vi "GroundStation final.vi"() -> ()   [LabVIEW 2022 SP3]
uses:
  <vilib>/Instr/_visa.llb/VISA Configure Serial Port (Instr).vi
  <vilib>/Utility/file.llb/Write Delimited Spreadsheet (string).vi
  <vilib>/picture/3D Picture Control/Object/Create Object (name).vi
  <vilib>/picture/3D Picture Control/Object/Add Object (no reference).vi
  <vilib>/picture/3D Picture Control/NI_3D Picture Control.lvlib
  <vilib>/httpClient/LabVIEWHTTPClient.lvlib
panel:
  out "Gas 3":string="Kg/M^3"
  out "Gas 2":dbl caption="Gas"
  out "X_axis 2":string
  out "Z_axis 2":string
  out "LiDAR_Read":string
  out "Angle":string
  out "Y_axis":string
  out "MPU 2":string
  out "GPS 3":string
  out "ANGLE Z":dbl
  out "ANGLE Y":dbl
  out "ANGLE X":dbl
  out "BMP 2":string
  out "MQ 2":string
  out "LIDAR":string
  out "Space":string
  out "DHT":string
  out "SPACE":string
  out "TEMP":string
  out "RH":string
  out "ALTITUDE":string
  out "PRESSURE":string
  out "GAS":string
  in  "Tab Control 2":enum32{"DASHBOARD", "SENSORS", "ABOUT"}(tab)
  out "Low Power":bool
  out "DHT":bool
  out "BMP":bool
  out "MQ":bool
  out "LIDAR":bool
  out "MPU":bool
  out "Pressure  2":dbl caption="Pressure"
  out "Pressure":string="Pascal"
  out "Altitude":string="Km/S^2"
  out "Altitude 2":dbl caption="Gas"
  out "Humidity":string="Km/S^2"
  out "rh":dbl caption="Humidity"
  out "Temp.":string="Celsius"
  out "Temperture 2":dbl caption="Temp"
  out "GPS":bool
  in  "Save Button":bool
  in  "Media Stop Button":bool
  in  "Play Button":bool
  out "System Status":string
  out "Battery Precentage":dbl format="%%%#_g"
  in  "Set Mode Button":bool
  in  "System Mode":T1(ring)
  in  "Save File Path":path
  in  "VISA resource name":refnum<visa-resource-name>
  in  "Save Button 2":bool
  out "Massage":string
  in  "Tab Control 4":T2(tab) caption="Tab Control 3"
  out "YAW":string
  out "PITCH":string
  out "ROLL":string
  out "Z MPU":string
  out "Y MPU":string
  out "X MPU":string
  in  "File Path":path
  in  "Apply Filter":bool
  out "Waveform Chart":dynamicdata(graph)
  out "3D Picture 2":refnum<vi>(3d-picture)
  out "z_axis":dbl
  out "Y_axis":dbl
  out "X_axis":dbl
  out "LIDAR_Read":dbl
  out "ANGLE":dbl
  out "XY Graph":cluster{"Y":dbl[], "Y":dbl[]}[](graph)
  out "Camera View":T3(plugin-control)
  in  "Stop Camera":bool
  in  "Start Camera":bool
  in  "Size Y":dbl
  in  "Size X":dbl
  in  "Zoom":dbl
  in  "Map Format":string(combo)
  in  "Character":string
  in  "Color":string
  in  "WebBrowser":refnum<k7>(container)
  out "LATITUDE":string
  out "LONGTUDE":string
  # "EARTH OBSERVATION SATELITE 2025"
  # "Power Management"
  # "Warnings"
  # "Live Sensors"
  # "Quick Actions"
  # "IMU & Orientation"
  # "This interface is part of a student project to develop a Ground Station for monitoring a CubeSat. It displays real-time sensor data, manages power modes, and streams live video from the satellite."
  # "Developed by:\n\n  Nevin Essam Helmy Gaber\n Youssif Ashraf \n\nAlong With the Team Members: \n\n Maged Micheal Seha     \n Abd-Elrahman Ramadan   \n Rawan Wael Elsayed   \n Bassam Khaled Eldawy  \n Marwa Gamal Hendawy    \n Yomna Saad Abd-Elazeem  \n Bavly Emil Tamer   \n Mostafa Mohamed Tawfik   \n Mariam Emadeldin Abdelrazik  \n Maryam Reda Elsayed   \n\nContact US:\n +201204037805"
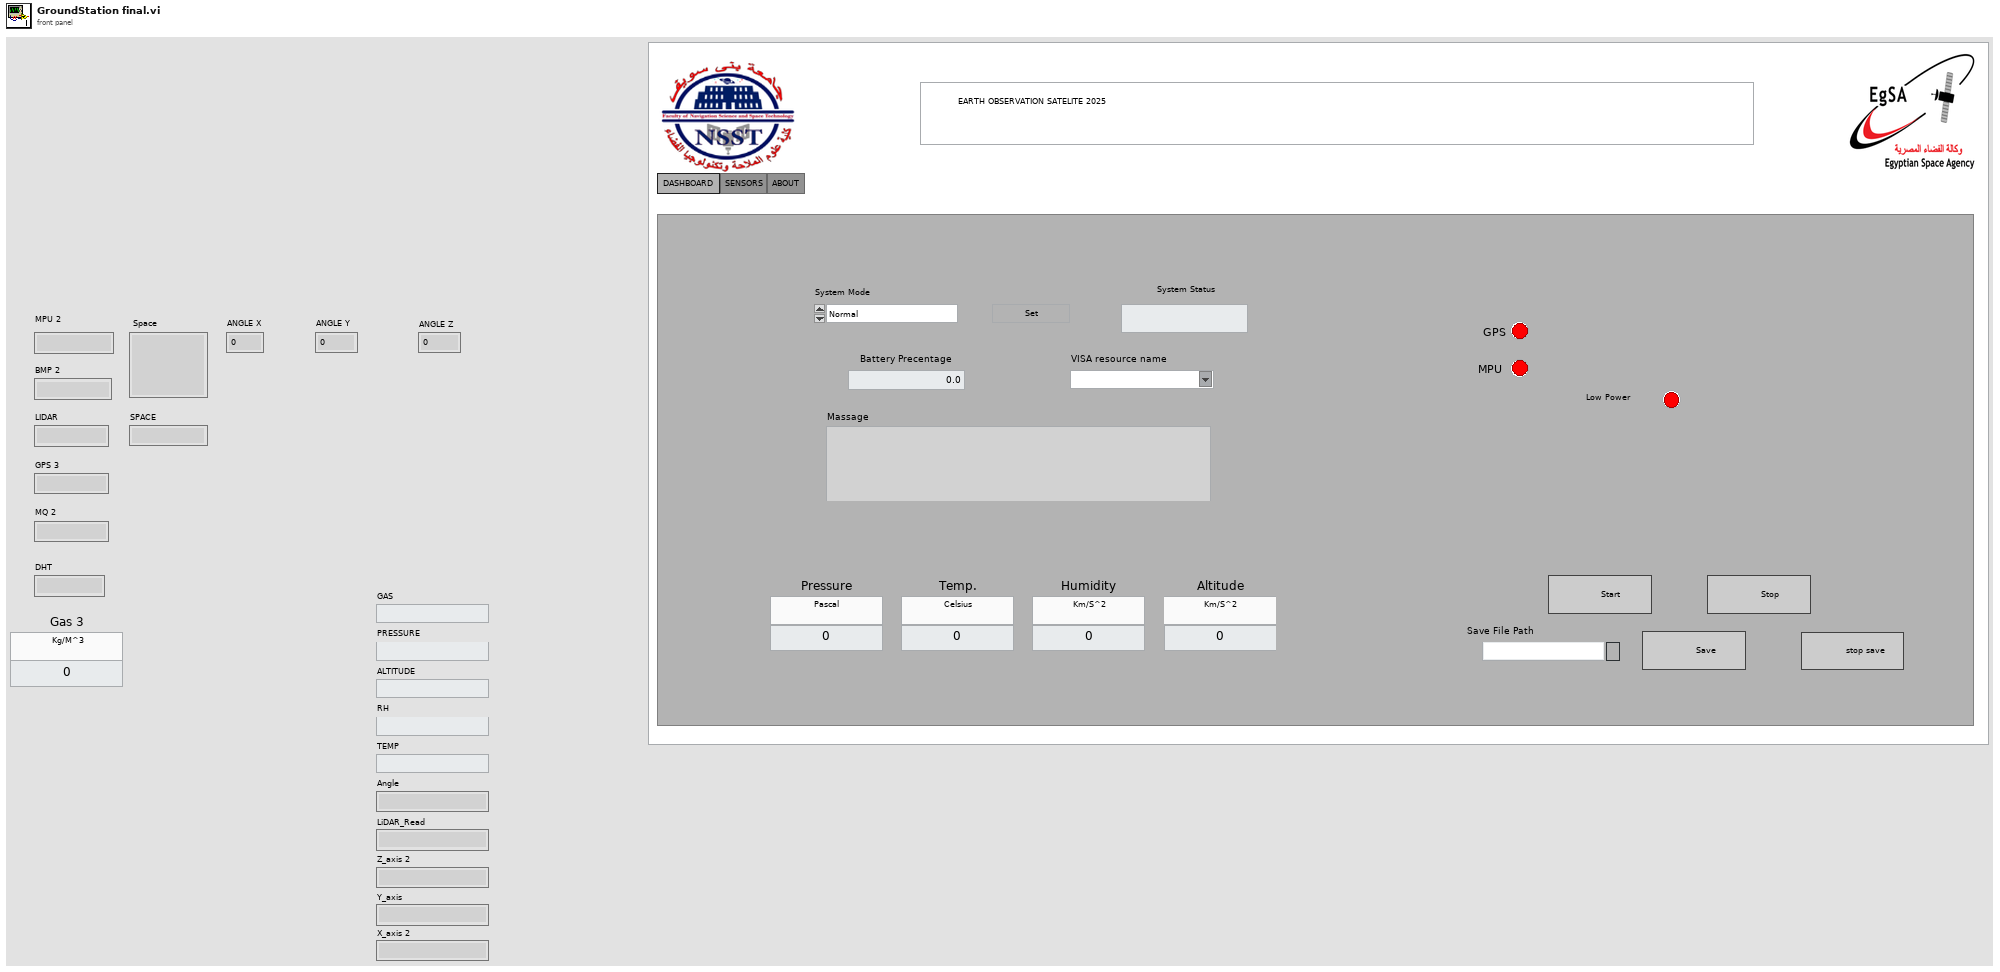
[diagram p1: front panel]
types:
  T1 = enum16{"Normal", "Power Saving", "Emergency", "Sleep"}
  T2 = enum32{"Sensors", "Sensors 2", "Ranging & Nav", "Vision & AI"}
  T3 = typedef "IMAQ Image.ctl" = refnum<image>
  T4 = typedef "Image Type" = u32
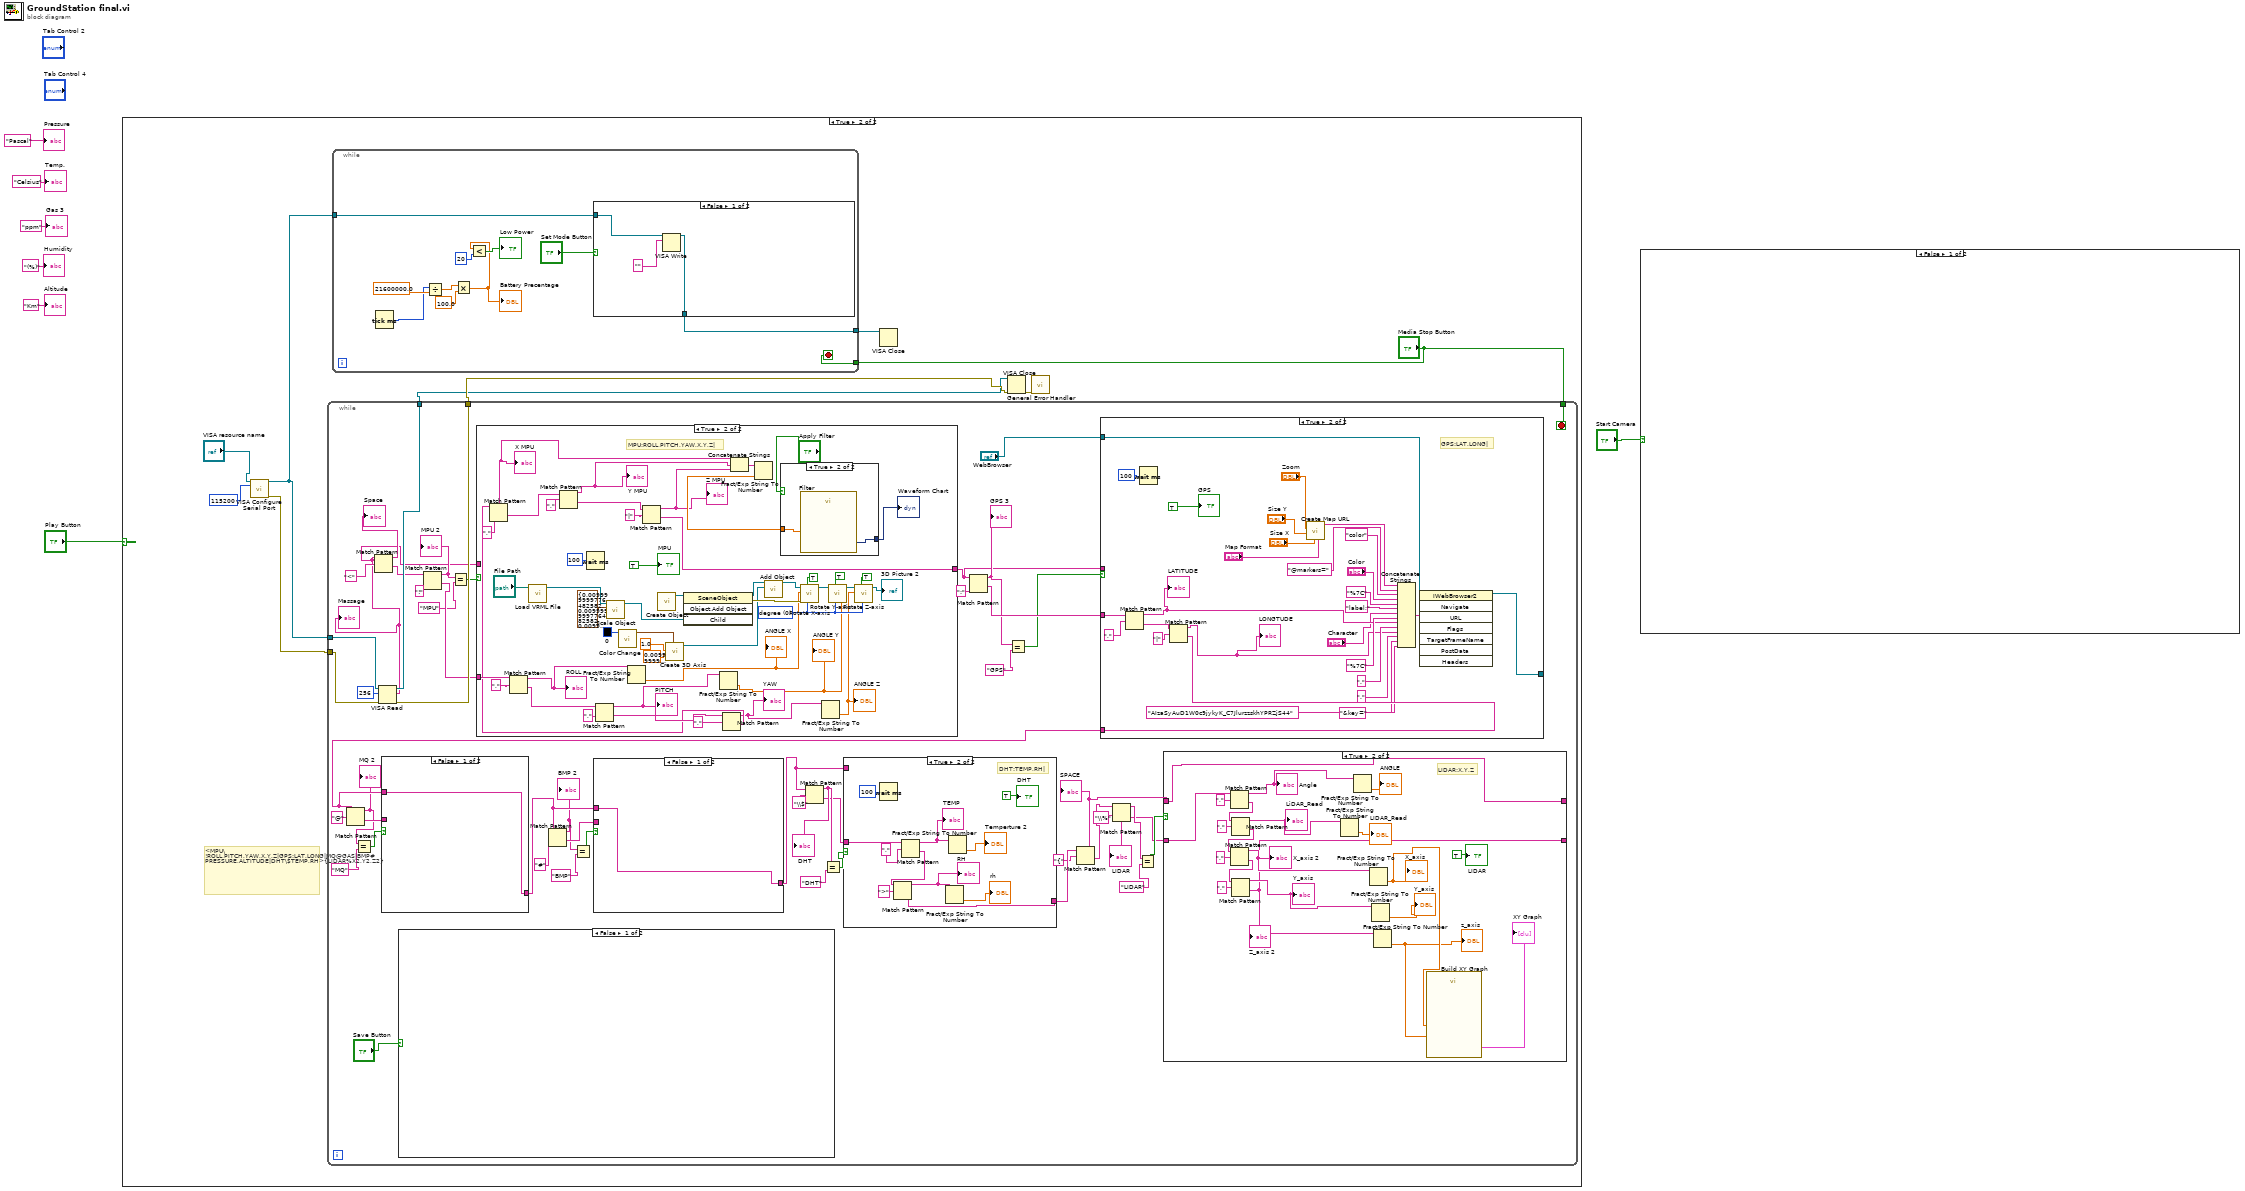
[diagram p0: block diagram]
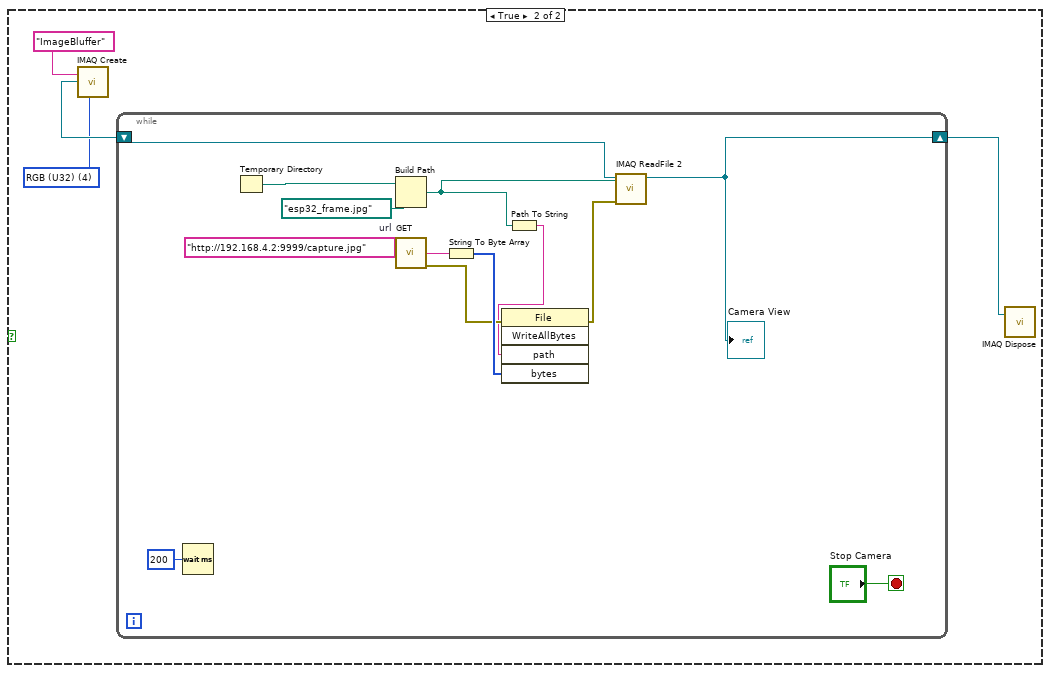
[diagram p2: hidden frame]
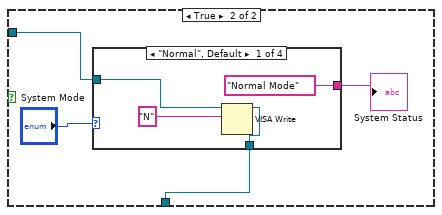
[diagram p4: hidden frame]
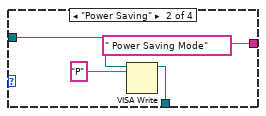
[diagram p5: hidden frame]
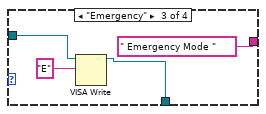
[diagram p6: hidden frame]
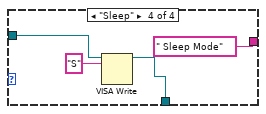
[diagram p7: hidden frame]
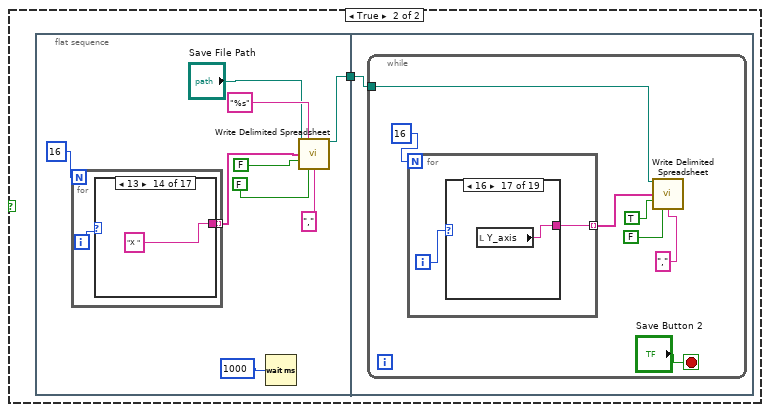
[diagram p8: hidden frame]
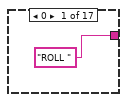
[diagram p9: hidden frame]
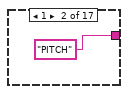
[diagram p10: hidden frame]
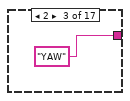
[diagram p11: hidden frame]
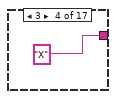
[diagram p12: hidden frame]
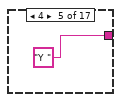
[diagram p13: hidden frame]
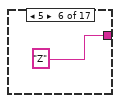
[diagram p14: hidden frame]
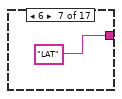
[diagram p15: hidden frame]
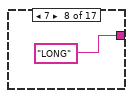
[diagram p16: hidden frame]
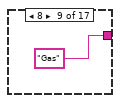
[diagram p17: hidden frame]
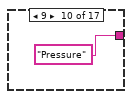
[diagram p18: hidden frame]
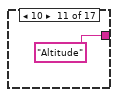
[diagram p19: hidden frame]
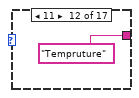
[diagram p20: hidden frame]
diagram:
  n1 = case shown="True" "Play Button" {
    frame False {
    }
    frame True {
      # "<MPU\\!ROLL,PITCH,YAW,X,Y,Z|GPS:LAT,LONG|MQ@GAS|BMP#PRESSURE,ALTITUDE|DHT\\$TEMP,RH>{LIDAR%X2,Y2,Z2}"
      n2 = call-poly "VISA Configure Serial Port"("VISA resource name"="VISA resource name", "baud rate (9600)"=u32 115200) -> ("VISA resource name out"=w9:refnum<visa-resource-name>, "error out"=w13:errorcluster)  [unwired: 12 in]
      n3 = while {
        tunnel: w9 -> [w100]
        tunnel: [w99] -> w15
        tunnel: w13 -> [w90]
        tunnel: [w91] -> w16
        tunnel: "Media Stop Button" -> [w59]
        stop <- w59 stop-if-true
        n4 = VISA Read(VISA resource name=w100, byte count=u32 256, error in (no error)=w90) -> (VISA resource name out=w99:refnum<visa-resource-name>, read buffer=w52:string, error out=w91:errorcluster)  [unwired: 1 out]
        "Massage" <- w52
        n5 = Match Pattern(string=w52, regular expression="<") -> (before substring=→"Space":string, after substring=w62:string)  [unwired: 1 in, 2 out]
        n6 = case shown="False" "Save Button" {
          frame False {
          }
          frame True {
            n7 = flat-sequence {
              tunnel: [w106] -> w101
              tunnel: w101 -> [w129]
              frame #0 {
                n8 = for {
                  N: 16 -> [_]
                  tunnel: [w111] -> w103 mode=indexing
                  i -> [w112]
                  n9 = case shown="13" w112 {
                    tunnel: ["ROLL " "PITCH" "YAW" "X" "Y " "Z" "LAT" "LONG" "Gas" "Pressure" "Altitude" "Tempruture" "RH " "X " "Y " "Z " _] -> w111
                    frame 0 {
                    }
                    frame 1 {
                    }
                    frame 2 {
                    }
                    frame 3 {
                    }
                    frame 4 {
                    }
                    frame 5 {
                    }
                    frame 6 {
                    }
                    frame 7 {
                    }
                    frame 8 {
                    }
                    frame 9 {
                    }
                    frame 10 {
                    }
                    frame 11 {
                    }
                    frame 12 {
                    }
                    frame 13 {
                    }
                    frame 14 {
                    }
                    frame 15 {
                    }
                    frame Default {
                    }
                  }
                }
                n10 = Wait (ms)(milliseconds to wait=u32 1000) -> ()  [unwired: 1 out]
                n11 = call-poly <vilib>:"Write Delimited Spreadsheet.vi"("file path (dialog if empty)"="Save File Path", "format (%s)"="%s" ("format (%.3f)"), "1D data"=w103, "append to file? (new file:F)"=FALSE, "transpose? (no:F)"=FALSE, "delimiter (\\t)"="," ("delimiter (\\t)")) -> ("new file path (Not A Path if cancelled)"=w106:path)  [unwired: 8 in, 1 out]
              }
              frame #1 {
                n12 = while {
                  tunnel: w129 -> [w132]
                  stop <- "Save Button 2" stop-if-true
                  n13 = for {
                    N: 16 -> [_]
                    tunnel: [w138] -> w131 mode=indexing
                    i -> [w137]
                    n14 = case shown="16" w137 {
                      tunnel: [w139 w140 w141 w142 w143 w144 w145 w146 w147 w148 w149 w150 w151 w152 w153 w154 w155 w156 _] -> w138
                      frame 0 {
                        n15 = local read "ROLL"() -> (w139:string)
                      }
                      frame 1 {
                        n16 = local read "PITCH"() -> (w140:string)
                      }
                      frame 2 {
                        n17 = local read "YAW"() -> (w141:string)
                      }
                      frame 3 {
                        n18 = local read "X MPU"() -> (w142:string)
                      }
                      frame 4 {
                        n19 = local read "Y MPU"() -> (w143:string)
                      }
                      frame 5 {
                        n20 = local read "Z MPU"() -> (w144:string)
                      }
                      frame 6 {
                        n21 = local read "LATITUDE"() -> (w145:string)
                      }
                      frame 7 {
                        n22 = local read "LONGTUDE"() -> (w146:string)
                      }
                      frame 8 {
                        n23 = local read "GAS"() -> (w147:string)
                      }
                      frame 9 {
                        n24 = local read "PRESSURE"() -> (w148:string)
                      }
                      frame 10 {
                        n25 = local read "ALTITUDE"() -> (w149:string)
                      }
                      frame 11 {
                        n26 = local read "TEMP"() -> (w150:string)
                      }
                      frame 12 {
                        n27 = local read "RH"() -> (w151:string)
                      }
                      frame 13 {
                        n28 = local read "Angle"() -> (w152:string)
                      }
                      frame 14 {
                        n29 = local read "LiDAR_Read"() -> (w153:string)
                      }
                      frame 15 {
                        n30 = local read "X_axis 2"() -> (w154:string)
                      }
                      frame 16 {
                        n31 = local read "Y_axis"() -> (w155:string)
                      }
                      frame 17 {
                        n32 = local read "Z_axis 2"() -> (w156:string)
                      }
                      frame 18, Default {
                      }
                    }
                  }
                  n33 = call-poly <vilib>:"Write Delimited Spreadsheet.vi"("file path (dialog if empty)"=w132, "1D data"=w131, "append to file? (new file:F)"=TRUE, "transpose? (no:F)"=FALSE, "delimiter (\\t)"="," ("delimiter (\\t)")) -> ()  [unwired: 9 in, 2 out]
                }
              }
            }
          }
        }
        n34 = Match Pattern(string=w62, regular expression="!") -> (before substring=w81:string, after substring=w89:string)  [unwired: 1 in, 2 out]
        "MPU 2" <- w81
        n35 = Equal?(x=w81, y="MPU") -> (x = y?=w83:bool)
        n36 = case shown="True" w83 {
          tunnel: w89 -> [_ w290]
          tunnel: [w242 w243] -> w51
          tunnel: w52 -> [w242 _]
          frame False {
          }
          frame True {
            w279 = u16 0 items=["degree", "radians"] ("angle unit")
            # "MPU:ROLL,PITCH,YAW,X,Y,Z|"
            n37 = Match Pattern(string=w290, regular expression=",") -> (before substring=w248:string, after substring=w261:string)  [unwired: 1 in, 2 out]
            "ROLL" <- w248
            n38 = call <vilib>:"Load VRML File.vi"("Path"="File Path") -> ("Scene:Read Scene File"=w265:refnum<vi>)  [unwired: 9 in, 1 out]
            n39 = Wait (ms)(milliseconds to wait=u32 100 ("millisecond timer value")) -> ()  [unwired: 1 out]
            n40 = Match Pattern(string=w261, regular expression=",") -> (before substring=w245:string, after substring=w260:string)  [unwired: 1 in, 2 out]
            "PITCH" <- w245
            n41 = call <vilib>:"Scale Object.vi"("Scale"=cluster{"X":sgl, "Y":sgl, "Z":sgl} {"X"=0.01, "Y"=0.01, "Z"=0.01}, "Scene.Object In"=w265) -> ("Scene.Object Out"=w264:refnum<vi>)  [unwired: 8 in, 1 out]
            n42 = call <vilib>:"Color Change.vi"("Color"=u32 0 ("Color Box")) -> ("RGBA"=w268:cluster{"R":sgl, "G":sgl, "B":sgl, "A":sgl})  [unwired: 10 in]
            n43 = Fract/Exp String To Number(string=w248) -> (number=w255:dbl)  [unwired: 3 in, 1 out]
            "ANGLE X" <- w255
            n44 = call-poly <vilib>:"Create Object.vi"() -> ("Scene:New Object"=w267:refnum<vi>)  [unwired: 10 in, 1 out]
            n45 = call <vilib>:"Create 3D Axis.vi"("Color"=w268, "Radius"=sgl 0.01, "Length"=sgl 1.0) -> ("New Object Refnum"=w283:refnum<vi>)  [unwired: 7 in, 1 out]
            n46 = invoke class="SceneObject" method="Object.Add Object"(reference=w267, "Child"=w264) -> (reference out=w284:refnum<vi>, error out=w288:errorcluster)  [unwired: 2 in, 2 out]
            n47 = Fract/Exp String To Number(string=w245) -> (number=w256:dbl)  [unwired: 3 in, 1 out]
            "ANGLE Y" <- w256
            n48 = Match Pattern(string=w260, regular expression=",") -> (before substring=w247:string, after substring=w259:string)  [unwired: 1 in, 2 out]
            "YAW" <- w247
            n49 = Match Pattern(string=w259, regular expression=",") -> (before substring=w254:string, after substring=w270:string)  [unwired: 1 in, 2 out]
            "X MPU" <- w254
            n50 = Match Pattern(string=w270, regular expression=",") -> (before substring=w244:string, after substring=w269:string)  [unwired: 1 in, 2 out]
            "Y MPU" <- w244
            n51 = Match Pattern(string=w269, regular expression="|") -> (before substring=w253:string, after substring=w243:string)  [unwired: 1 in, 2 out]
            "Z MPU" <- w253
            n52 = Concatenate Strings(w254, w244, w253) -> (w263:string)
            n53 = Fract/Exp String To Number(string=w263) -> (number=w289:dbl)  [unwired: 3 in, 1 out]
            n54 = call-poly <vilib>:"Add Object.vi"("New Object In"=w283, "Scene Object In"=w284) -> ("Scene Object Out"=w282:refnum<vi>)  [unwired: 8 in, 1 out]
            n55 = case shown="True" "Apply Filter" {
              tunnel: w289 -> [_ w292]
              tunnel: [w291 w293] -> w252
              frame False {
                n56 = call "Convert to Dynamic Data"() -> ("Dynamic Data Type"=w291:dynamicdata)  [unwired: 4 in]
              }
              frame True {
                n57 = call "Filter"("Signal"=w292) -> ("Filtered Signal"=w293:dynamicdata)  [unwired: 9 in, 1 out]
              }
            }
            "Waveform Chart" <- w252
            n58 = call <vilib>:"Rotate X-axis.vi"("angle unit"=w279, "Relative?"=TRUE, "error in (no error)"=w288, "angle"=w255, "Scene Object In"=w282) -> ("Scene Object Out"=w281:refnum<vi>)  [unwired: 5 in, 1 out]
            n59 = Fract/Exp String To Number(string=w247) -> (number=w257:dbl)  [unwired: 3 in, 1 out]
            "ANGLE Z" <- w257
            n60 = call <vilib>:"Rotate Y-axis.vi"("angle unit"=w279, "Relative?"=TRUE, "angle"=w256, "Scene Object In"=w281) -> ("Scene Object Out"=w280:refnum<vi>)  [unwired: 6 in, 1 out]
            n61 = call <vilib>:"Rotate Z-axis.vi"("angle unit"=w279, "Relative?"=TRUE, "angle"=w257, "Scene Object In"=w280) -> ("Scene Object Out"=→"3D Picture 2":refnum<vi>)  [unwired: 6 in, 1 out]
            "MPU" <- TRUE
          }
        }
        n62 = Match Pattern(string=w51, regular expression=":") -> (before substring=w79:string, after substring=w88:string)  [unwired: 1 in, 2 out]
        "GPS 3" <- w79
        n63 = Equal?(x=w79, y="GPS") -> (x = y?=w78:bool)
        n64 = case shown="True" w78 {
          tunnel: "WebBrowser" -> [w213 w241]
          tunnel: [w212 w240] -> w84
          tunnel: w88 -> [_ w239]
          tunnel: [w213 w223] -> _
          tunnel: w51 -> [w212 _]
          frame False {
          }
          frame True {
            # "GPS:LAT,LONG|"
            n65 = Match Pattern(string=w239, regular expression=",") -> (before substring=w221:string, after substring=w225:string)  [unwired: 1 in, 2 out]
            "LATITUDE" <- w221
            n66 = Wait (ms)(milliseconds to wait=u32 100) -> ()  [unwired: 1 out]
            n67 = Match Pattern(string=w225, regular expression="|") -> (before substring=w220:string, after substring=w240:string)  [unwired: 1 in, 2 out]
            "LONGTUDE" <- w220
            n68 = call "Create Map URL.vi"("Map Format"="Map Format", "X"="Size X", "Y"="Size Y", "Zoom"="Zoom") -> ("String"=w238:string)  [unwired: 7 in]
            n69 = Concatenate Strings(w238, "@markers=" ("string"), "color" ("string"), "Color", "%7C" ("string"), "label;" ("string"), "Character", "%7C" ("string"), w221, "." ("string"), w220, "." ("string"), "&key=" ("string"), "AIzaSyAuD1W0c9jykyK_C7JlurzzskhYPRZjS44" ("string")) -> (w232:string)
            n70 = invoke class="IWebBrowser2" method="Navigate"(reference=w241, "URL"=w232) -> (reference out=w223:refnum<k7>)  [unwired: 6 in, 7 out]
            "GPS" <- TRUE
          }
        }
        n71 = Match Pattern(string=w84, regular expression="@") -> (before substring=w76:string, after substring=w87:string)  [unwired: 1 in, 2 out]
        "MQ 2" <- w76
        n72 = Equal?(x=w76, y="MQ") -> (x = y?=w75:bool)
        n73 = case shown="False" w75 {
          tunnel: w87 -> [_ w211]
          tunnel: [w204 w210] -> w85
          tunnel: w84 -> [w204 _]
          frame False {
          }
          frame True {
            # "MQ:GAS|"
            n74 = Match Pattern(string=w211, regular expression="|") -> (before substring=w205:string, after substring=w210:string)  [unwired: 1 in, 2 out]
            "GAS" <- w205
            n75 = Wait (ms)(milliseconds to wait=u32 100) -> ()  [unwired: 1 out]
            n76 = Fract/Exp String To Number(string=w205) -> (number=→"Gas 2":dbl)  [unwired: 3 in, 1 out]
            "MQ" <- TRUE
          }
        }
        n77 = Match Pattern(string=w85, regular expression="#") -> (before substring=w73:string, after substring=w86:string)  [unwired: 1 in, 2 out]
        "BMP 2" <- w73
        n78 = Equal?(x=w73, y="BMP") -> (x = y?=w72:bool)
        n79 = case shown="False" w72 {
          tunnel: [w192 w203] -> w64
          tunnel: w86 -> [_ w202]
          tunnel: w85 -> [w192 _]
          frame False {
          }
          frame True {
            # "BMP:PRESSURE,ALTITUDE|"
            n80 = Wait (ms)(milliseconds to wait=u32 100) -> ()  [unwired: 1 out]
            n81 = Match Pattern(string=w202, regular expression=",") -> (before substring=w196:string, after substring=w198:string)  [unwired: 1 in, 2 out]
            "PRESSURE" <- w196
            n82 = Match Pattern(string=w198, regular expression="|") -> (before substring=w194:string, after substring=w203:string)  [unwired: 1 in, 2 out]
            "ALTITUDE" <- w194
            n83 = Fract/Exp String To Number(string=w196) -> (number=→"Pressure  2":dbl)  [unwired: 3 in, 1 out]
            n84 = Fract/Exp String To Number(string=w194) -> (number=→"Altitude 2":dbl)  [unwired: 3 in, 1 out]
            "BMP" <- TRUE
          }
        }
        n85 = Match Pattern(string=w64, regular expression="\\$") -> (before substring=w66:string, after substring=w65:string)  [unwired: 1 in, 2 out]
        "DHT" <- w66
        n86 = Equal?(x=w66, y="DHT") -> (x = y?=w70:bool)
        n87 = case shown="True" w70 {
          tunnel: w65 -> [_ w191]
          tunnel: [w180 w190] -> w61
          tunnel: w64 -> [w180 _]
          frame False {
          }
          frame True {
            # "DHT:TEMP,RH|"
            n88 = Wait (ms)(milliseconds to wait=u32 100) -> ()  [unwired: 1 out]
            n89 = Match Pattern(string=w191, regular expression=",") -> (before substring=w183:string, after substring=w186:string)  [unwired: 1 in, 2 out]
            "TEMP" <- w183
            n90 = Match Pattern(string=w186, regular expression=">") -> (before substring=w181:string, after substring=w190:string)  [unwired: 1 in, 2 out]
            "RH" <- w181
            n91 = Fract/Exp String To Number(string=w181) -> (number=→"rh":dbl)  [unwired: 3 in, 1 out]
            n92 = Fract/Exp String To Number(string=w183) -> (number=→"Temperture 2":dbl)  [unwired: 3 in, 1 out]
            "DHT" <- TRUE
          }
        }
        n93 = Match Pattern(string=w61, regular expression="{") -> (before substring=w54:string, after substring=w55:string)  [unwired: 1 in, 2 out]
        "SPACE" <- w54
        n94 = Match Pattern(string=w55, regular expression="\\%") -> (before substring=w68:string, after substring=w56:string)  [unwired: 1 in, 2 out]
        "LIDAR" <- w68
        n95 = Equal?(x=w68, y="LIDAR") -> (x = y?=w67:bool)
        n96 = case shown="True" w67 {
          tunnel: w56 -> [w157 w171]
          tunnel: [w158 w163] -> _
          tunnel: w54 -> [w158 w163]
          tunnel: [w157 w164] -> _
          frame False {
          }
          frame True {
            # "LIDAR:X,Y,Z"
            n97 = Match Pattern(string=w171, regular expression=",") -> (before substring=w170:string, after substring=w174:string)  [unwired: 1 in, 2 out]
            "Angle" <- w170
            n98 = Match Pattern(string=w174, regular expression=",") -> (before substring=w168:string, after substring=w172:string)  [unwired: 1 in, 2 out]
            "LiDAR_Read" <- w168
            n99 = Match Pattern(string=w172, regular expression=",") -> (before substring=w167:string, after substring=w173:string)  [unwired: 1 in, 2 out]
            "X_axis 2" <- w167
            n100 = Match Pattern(string=w173, regular expression=",") -> (before substring=w165:string, after substring=w164:string)  [unwired: 1 in, 2 out]
            "Y_axis" <- w165
            "Z_axis 2" <- w164
            n101 = Fract/Exp String To Number(string=w168) -> (number=→"LIDAR_Read":dbl)  [unwired: 3 in, 1 out]
            n102 = Fract/Exp String To Number(string=w170) -> (number=→"ANGLE":dbl)  [unwired: 3 in, 1 out]
            n103 = Fract/Exp String To Number(string=w167) -> (number=w160:dbl)  [unwired: 3 in, 1 out]
            "X_axis" <- w160
            n104 = Fract/Exp String To Number(string=w165) -> (number=→"Y_axis":dbl)  [unwired: 3 in, 1 out]
            n105 = Fract/Exp String To Number(string=w164) -> (number=w159:dbl)  [unwired: 3 in, 1 out]
            "z_axis" <- w159
            n106 = call "Build XY Graph"("Y Input"=w159, "X Input"=w160) -> ("XY Graph"=→"XY Graph":cluster{"X":dbl[], "Y":dbl[]}[])  [unwired: 8 in, 1 out]
            "LIDAR" <- TRUE
          }
        }
      }
      n107 = while {
        tunnel: "Media Stop Button" -> [w24]
        tunnel: w9 -> [w23]
        tunnel: [w18] -> w8
        stop <- w24 stop-if-true
        n108 = Tick Count (ms)() -> (millisecond timer value=w17:u32)
        n109 = Divide(x=w17, y=21600000.0) -> (x/y=w21:dbl)
        n110 = Multiply(x=w21, y=100.0) -> (x*y=w19:dbl)
        "Battery Precentage" <- w19
        n111 = Less?(x=w19, y=20) -> (x < y?=→"Low Power":bool)
        n112 = case shown="False" "Set Mode Button" {
          tunnel: w23 -> [w29 w32]
          tunnel: [w28 w31] -> w18
          frame False {
            n113 = VISA Write(VISA resource name=w29, write buffer="") -> (VISA resource name out=w28:refnum<visa-resource-name>)  [unwired: 1 in, 2 out]
          }
          frame True {
            n114 = case shown="\"Normal\", Default" "System Mode" {
              tunnel: ["Normal Mode" " Power Saving Mode" " Emergency Mode " " Sleep Mode"] -> w33
              tunnel: w32 -> [w36 w40 w44 w48]
              tunnel: [w35 w39 w43 w47] -> w31
              frame "Normal", Default {
                n115 = VISA Write(VISA resource name=w36, write buffer="N") -> (VISA resource name out=w35:refnum<visa-resource-name>)  [unwired: 1 in, 2 out]
              }
              frame "Power Saving" {
                n116 = VISA Write(VISA resource name=w40, write buffer="P") -> (VISA resource name out=w39:refnum<visa-resource-name>)  [unwired: 1 in, 2 out]
              }
              frame "Emergency" {
                n117 = VISA Write(VISA resource name=w44, write buffer="E") -> (VISA resource name out=w43:refnum<visa-resource-name>)  [unwired: 1 in, 2 out]
              }
              frame "Sleep" {
                n118 = VISA Write(VISA resource name=w48, write buffer="S") -> (VISA resource name out=w47:refnum<visa-resource-name>)  [unwired: 1 in, 2 out]
              }
            }
            "System Status" <- w33
          }
        }
      }
      n119 = VISA Close(VISA resource name=w8) -> ()  [unwired: 1 in, 1 out]
      n120 = VISA Close(VISA resource name=w15, error in (no error)=w16) -> (error out=w14:errorcluster)
      n121 = call <vilib>:"General Error Handler.vi"("error in (no error)"=w14) -> ()  [unwired: 10 in, 5 out]
    }
  }
  n122 = case shown="False" "Start Camera" {
    frame False {
    }
    frame True {
      w295 = T4 4 items=["Grayscale (U8)", "Grayscale (I16)", "Grayscale (SGL)", "Complex (CSG)", "RGB (U32)", "HSL (U32)", "RGB (U64)", "Grayscale (U16)"] ("Image Type")
      n123 = call "IMAQ Create"("Image Name"="ImageBluffer", "Image Type"=w295) -> ("New Image"=w296:T3)  [unwired: 3 in, 1 out]
      n124 = while {
        shift-right: [w299] -> w294
        shift-left: w296 -> [w309]
        stop <- "Stop Camera" stop-if-true
        w310 = "http://192.168.4.2:9999/capture.jpg"  # url
        n125 = Wait (ms)(milliseconds to wait=u32 200) -> ()  [unwired: 1 out]
        n126 = Temporary Directory() -> (w308:path)
        n127 = Build Path(base path=w308, name or relative path=path "esp32_frame.jpg") -> (appended path=w301:path)
        n128 = call <vilib>:"GET.vi"("url"=w310) -> ("body"=w305:string, "error out"=w303:errorcluster)  [unwired: 11 in, 2 out]
        n129 = String To Byte Array(string=w305) -> (unsigned byte array=w304:u8[])
        n130 = Path To String(path=w301) -> (string=w300:string)
        n131 = invoke class="File" method="WriteAllBytes"(error in=w303, "path"=w300, "bytes"=w304) -> (error out=w302:errorcluster)  [unwired: 2 in, 4 out]
        n132 = call "IMAQ ReadFile 2"("File Path"=w301, "error in (no error)"=w302, "Image"=w309) -> ("Image Out"=w299:T3)  [unwired: 4 in, 4 out]
        "Camera View" <- w299
      }
      n133 = call "IMAQ Dispose"("Image"=w294) -> ()  [unwired: 5 in, 1 out]
    }
  }
  "Pressure" <- "Pascal" ("Pressure")
  "Temp." <- "Celsius" ("Temp.")
  "Gas 3" <- "ppm" ("Gas")
  "Humidity" <- "(%)" ("Humidity")
  "Altitude" <- "Km" ("Altitude")
